vi "AWSEXE.vi"(8 "error in (no error)":errorcluster, 9 "New/Old(T)":bool, 10 "RX/RY":string, 11 "DUT":string) -> (0 "error in (out)":errorcluster, 2 "Result":string)   [LabVIEW 2024, in "AWSEXE.lvlib"]
doc: "This template is for the Queued Message Handler design pattern.\n\nThe Event Handling Loop generates messages based on user interface actions.\n\nThe Message Handling Loop processes messages generated by the Event Handling Loop, or by other messages. The messages are string values, so new messages can be added easily to the Message Cases case structure in the Message Handling Loop. Each message cluster can also provide an optional value for Message Data, which is a variant that can be converted to whatever message-specific data is required."
uses:
  AWSEXE.lvlib
  support/Neoway_ctrl.ctl
  controls/Neoway UI Data.ctl
  PrivateControls/FGV_Queue_Control.ctl
  <vilib>/Utility/error.llb/Error Cluster From Error Code.vi
  <vilib>/ErrorRing/Error Ring.xnode
  support/Message Queue/Neoway Message Queue.lvlib
  support/User Event - Stop/72-13360 User Event - Stop.lvlib
  Launcher/Launcher_DTU.lvlib
panel:
  in  "Neoway Flashing":T1
  in  "Config":string
  in  "Read_Res":bool
  in  "Read_Current":bool
  in  "Read_File":bool
  in  "Flash":bool
  out "queue name 2":string
  out "queue name":string
  out "Display <Replace Me>":string
  in  "Output":bool
  in  "Init_Neoway":bool
  in  "Exit":bool
  # "These controls have associated \"Value Changed\" events configured in the Event Structure on the diagram.\n\nReplace them (and reconfigure the Event Structure) with the controls you need for your application."
  # "This template is for the Queued Message Handler design pattern.\n\nSee the block diagram for more information on how to use this template."
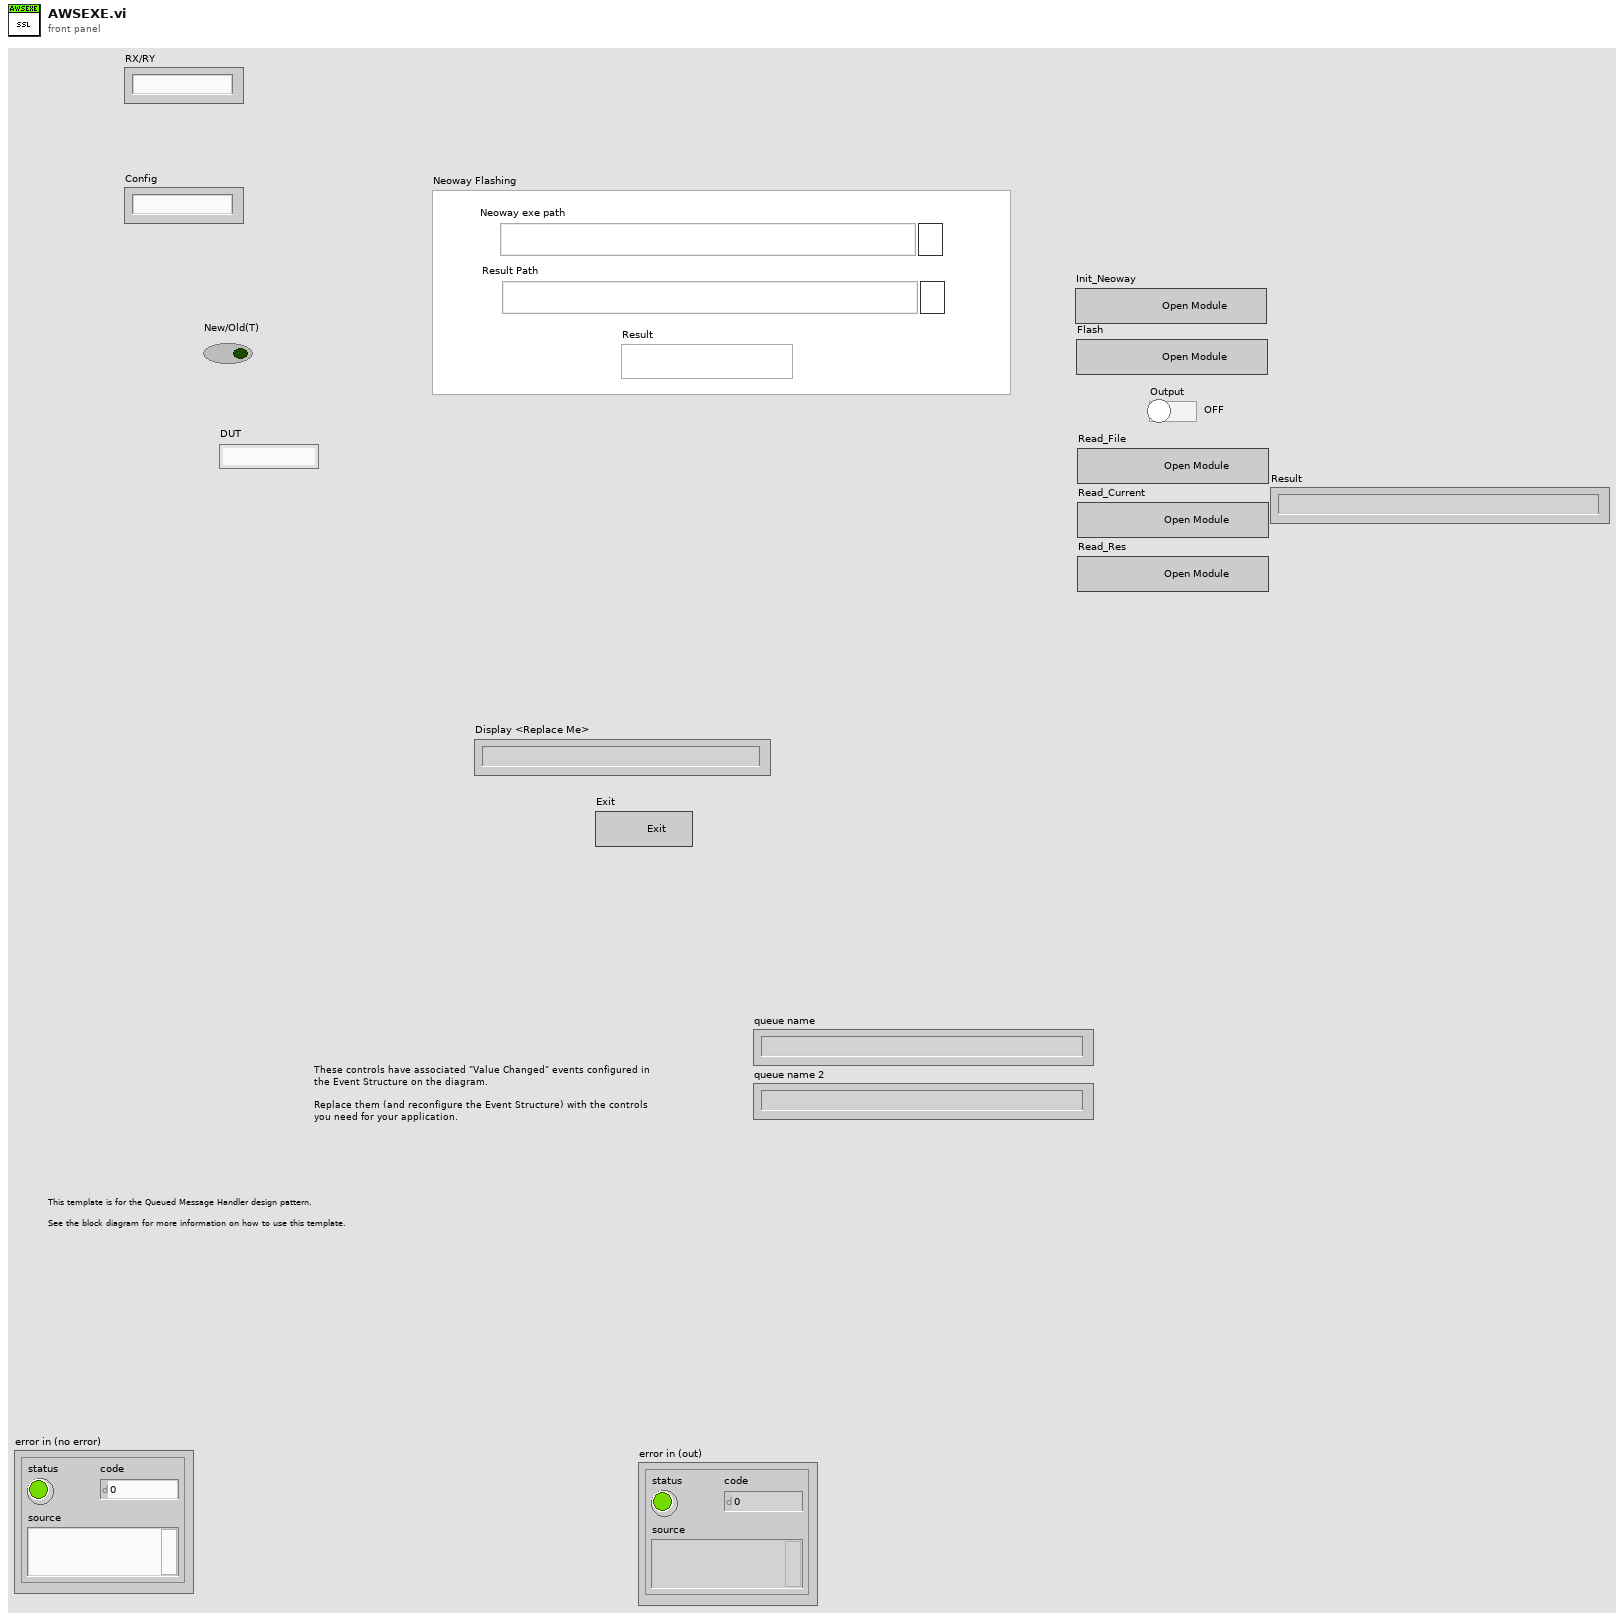
[diagram p1: front panel]
types:
  T1 = typedef "AWSEXE.lvlib/Neoway_ctrl.ctl" = cluster{"Neoway exe path":path, "Result Path":path, "Result":string}
  T2 = typedef "AWSEXE.lvlib/Neoway UI Data.ctl" = cluster{"DUT":string, "Neoway_Q":refnum<queue>, "notifier out":refnum<notifier>, "Config":string, "Neoway Flashing":T1, "Bat file path":path, "Exe path":string, "Flash path":string, "Result":string, "Timer":u32}
  T3 = typedef "AWSEXE.lvlib/FGV_Queue_Control.ctl" = enum16{"Release", "Get", "Set"}
  T4 = typedef "AWSEXE.lvlib/Neoway Message Queue.lvlib/All Message Queues.ctl" = cluster{"UI":refnum<queue>, "QSM":refnum<queue>}
  T5 = cluster{"Message":string, "Message Data":variant}
  T6 = enum16{"Read", "Write", "All_sections", "All_values", "Remove key&section"}
  T7 = enum16{"open", "replace", "create", "open or create", "replace or create", "replace or create with confirmation"}
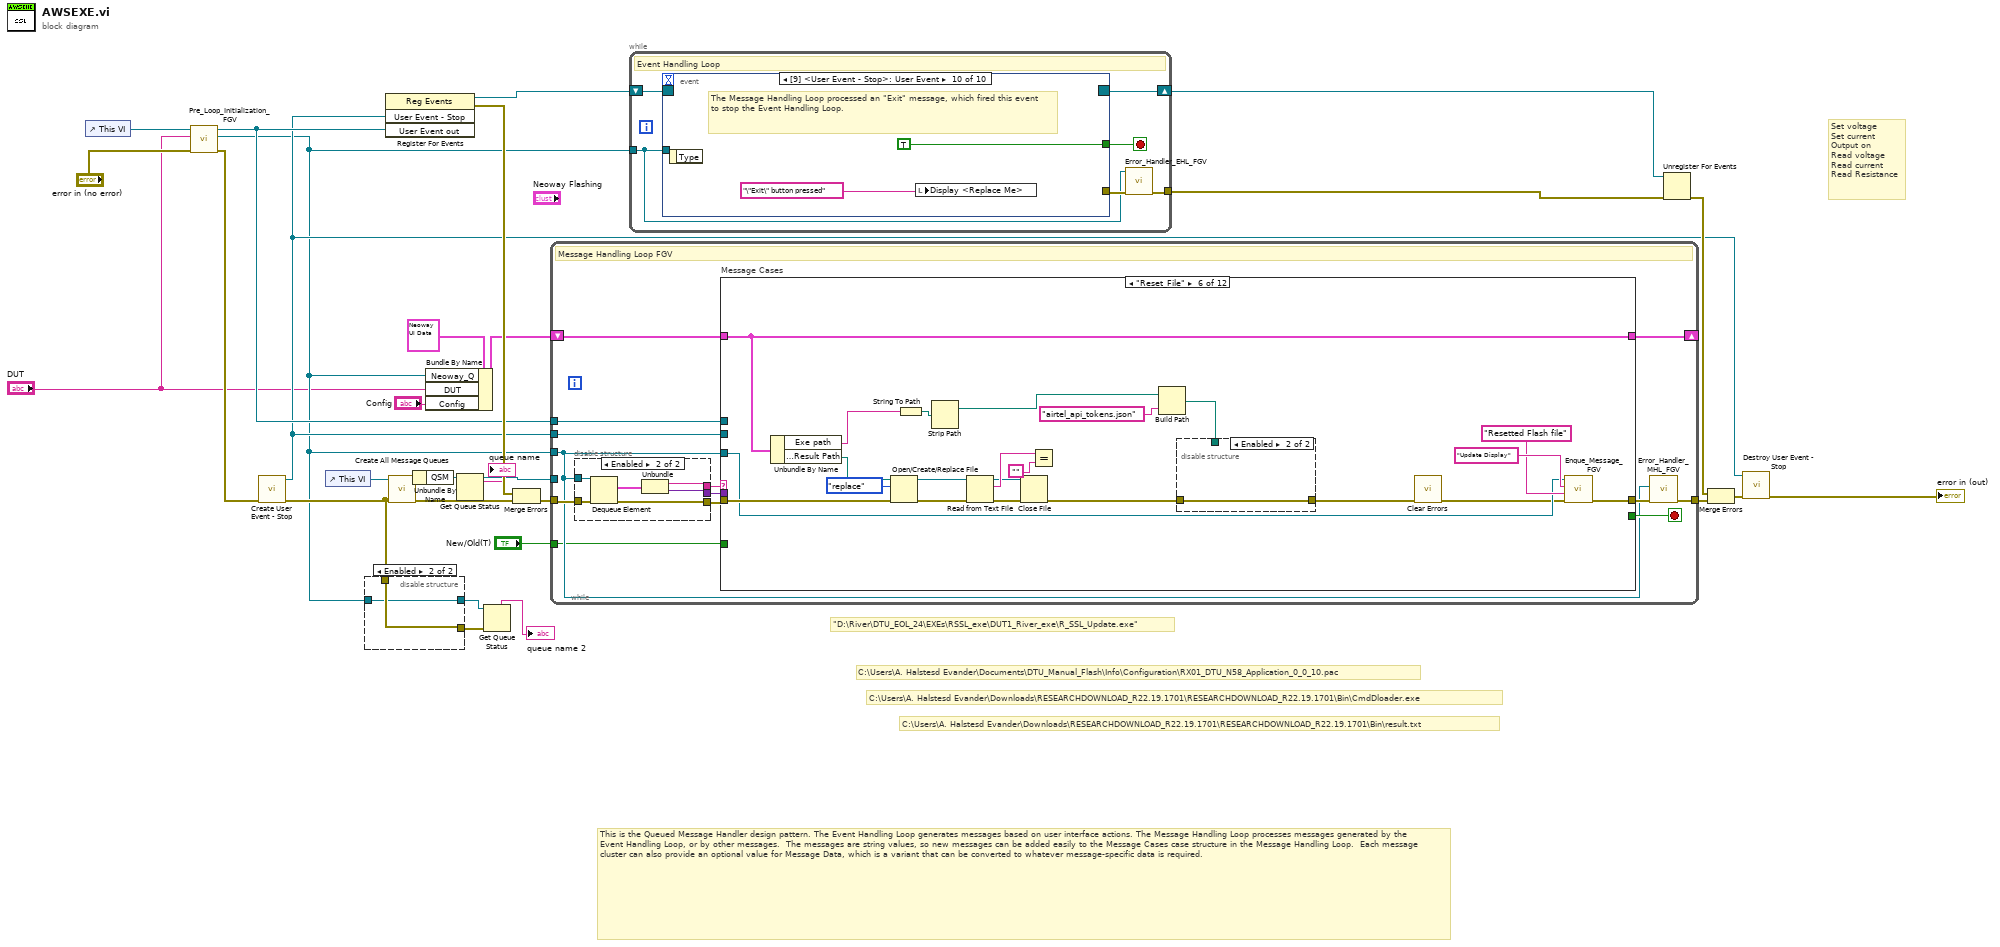
[diagram p0: block diagram]
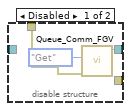
[diagram p2: hidden frame]
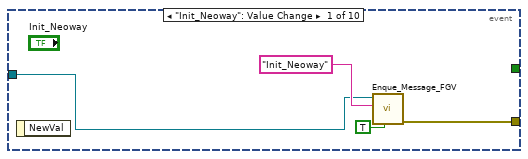
[diagram p3: hidden frame]
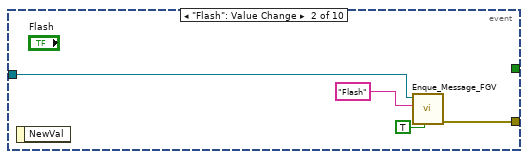
[diagram p4: hidden frame]
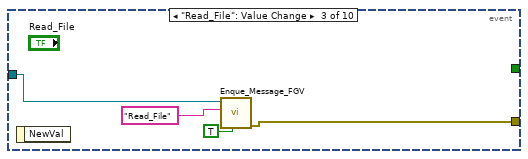
[diagram p5: hidden frame]
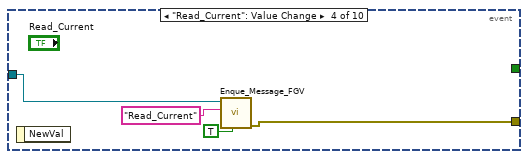
[diagram p6: hidden frame]
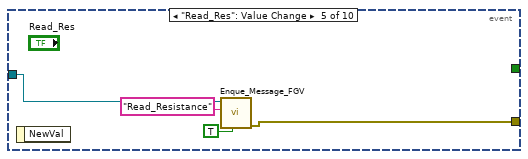
[diagram p7: hidden frame]
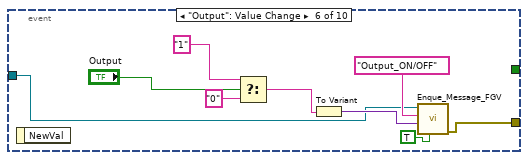
[diagram p8: hidden frame]
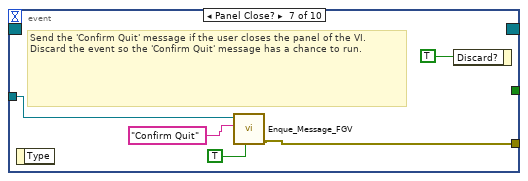
[diagram p9: hidden frame]
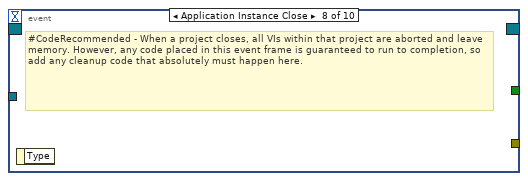
[diagram p10: hidden frame]
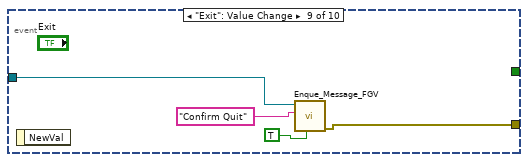
[diagram p11: hidden frame]
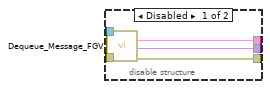
[diagram p12: hidden frame]
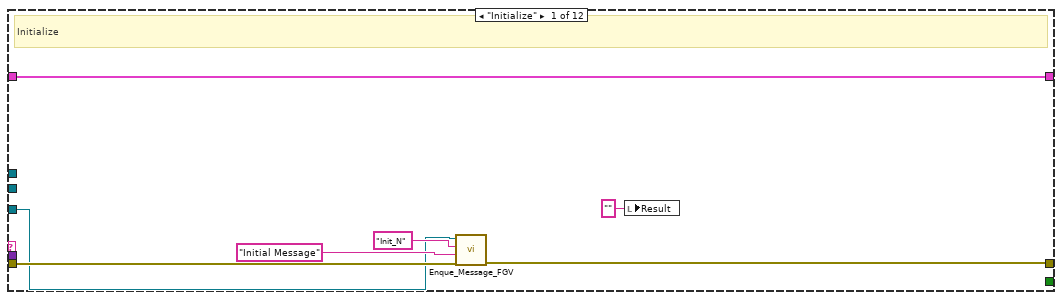
[diagram p13: hidden frame]
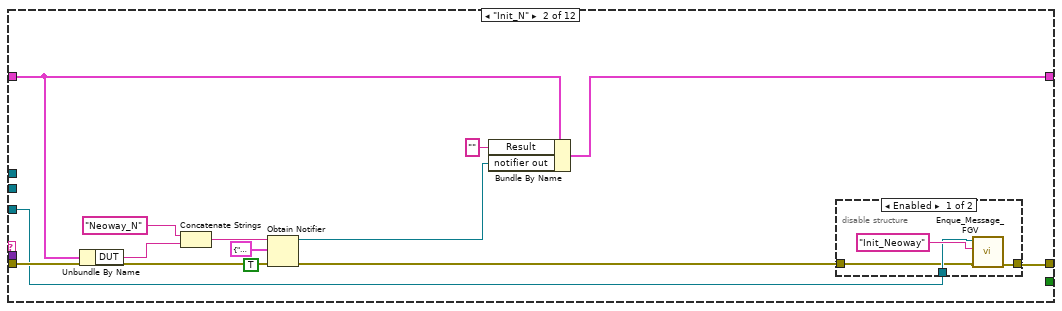
[diagram p14: hidden frame]
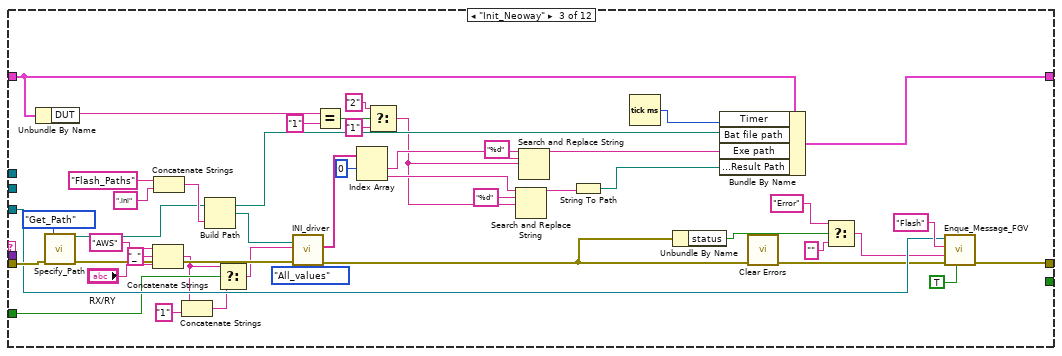
[diagram p16: hidden frame]
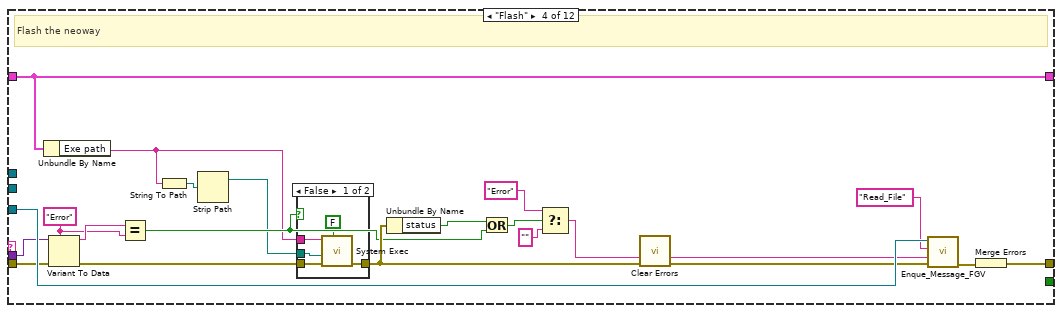
[diagram p17: hidden frame]
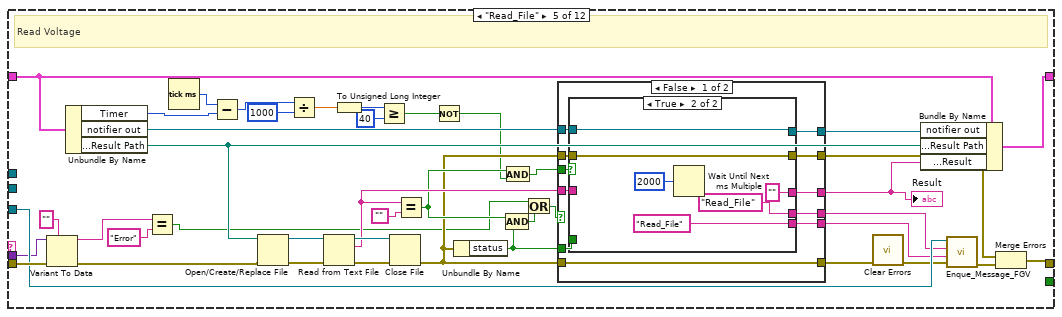
[diagram p19: hidden frame]
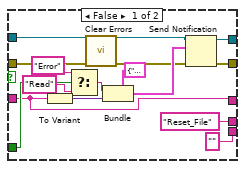
[diagram p20: hidden frame]
diagram:
  # "\"D:\\River\\DTU_EOL_24\\EXEs\\RSSL_exe\\DUT1_River_exe\\R_SSL_Update.exe\""
  # "C:\\Users\\A. Halstesd Evander\\Downloads\\RESEARCHDOWNLOAD_R22.19.1701\\RESEARCHDOWNLOAD_R22.19.1701\\Bin\\result.txt"
  # "C:\\Users\\A. Halstesd Evander\\Downloads\\RESEARCHDOWNLOAD_R22.19.1701\\RESEARCHDOWNLOAD_R22.19.1701\\Bin\\CmdDloader.exe"
  # "C:\\Users\\A. Halstesd Evander\\Documents\\DTU_Manual_Flash\\Info\\Configuration\\RX01_DTU_N58_Application_0_0_10.pac"
  # "Set voltage\nSet current\nOutput on\nRead voltage \nRead current\nRead Resistance"
  # "This is the Queued Message Handler design pattern. The Event Handling Loop generates messages based on user interface actions. The Message Handling Loop processes messages generated by the Event Handling Loop, or by other messages.  The messages are string values, so new messages can be added easily to the Message Cases case structure in the Message Handling Loop.  Each message cluster can also provide an optional value for Message Data, which is a variant that can be converted to whatever message-specific data is required."
  n1 = control-ref of="This VI"() -> (w18:refnum<vi>)
  n2 = call "Pre_Loop_Initialization_FGV.vi"("error in (no error)"="error in (no error)", "DUT"="DUT", "VI in"=w18) -> ("error out"=w16:errorcluster, "queue out"=w4:refnum<queue>, "User Event out"=w8:refnum<user-event>)  [unwired: 6 in]
  n3 = call "Create User Event - Stop.vi"("error in (no error)"=w16) -> ("error out"=w11:errorcluster, "User Event - Stop"=w7:refnum<user-event>)  [unwired: 9 in]
  n4 = control-ref of="This VI"() -> (w14:refnum<vi>)
  n5 = disable-structure shown="Enabled" {
    disable-tunnel: w11 -> [w33 w35]
    disable-tunnel: [w31 w34] -> w10
    disable-tunnel: [_ w35] -> w6
    disable-tunnel: w4 -> [_ w34]
    frame Disabled {
      n6 = call "Queue_Comm_FGV.vi"("error in (no error)"=w33, "Enum"=FGV_Queue_Control."Get") -> ("queue Out"=w31:refnum<queue>)  [unwired: 8 in, 1 out]
    }
    frame Enabled {
    }
  }
  n7 = register-events(w7, w8) -> (reference out=w21:refnum<event-registration>, error out=w19:errorcluster)  [unwired: 2 in]
  n8 = call "Create All Message Queues.vi"("error in (no error)"=w11, "This VI"=w14) -> ("error out"=w30:errorcluster, "Message Queues out"=w29:T4)  [unwired: 8 in]
  n9 = Unbundle By Name(w29) -> ("QSM"=w27:refnum<queue>)
  n10 = Bundle By Name(cluster=T2 {"DUT"="", "Neoway_Q"=refnum, "notifier out"=refnum, "Config"="", "Neoway Flashing"={"Neoway exe path"=path "", "Result Path"=path "", "Result"=""}, "Bat file path"=path "", "Exe path"="", "Flash path"="", "Result"="", "Timer"=0} ("Data Cluster"), "Neoway_Q"=w4, "DUT"="DUT", "Config"="Config") -> (w5:T2)
  n11 = Get Queue Status(queue=w27) -> (queue out=w13:refnum<queue>, queue name=→"queue name":string)  [unwired: 2 in, 6 out]
  n12 = Get Queue Status(queue=w10, error in (no error)=w6) -> (queue name=→"queue name 2":string)  [unwired: 1 in, 7 out]
  n13 = Merge Errors(w19, w30) -> (w20:errorcluster)
  n14 = while {
    tunnel: w13 -> [_]
    shift-right: [w47] -> _
    shift-left: w5 -> [w48]
    tunnel: w8 -> [w45]
    tunnel: w20 -> [w44]
    tunnel: [w39] -> w28
    tunnel: w7 -> [w38]
    tunnel: w4 -> [w37]
    tunnel: "New/Old(T)" -> [w36]
    stop <- w46 stop-if-true
    # "Message Handling Loop FGV"
    n15 = disable-structure shown="Enabled" {
      disable-tunnel: w44 -> [w52 w58]
      disable-tunnel: [w51 w56] -> w43
      disable-tunnel: [w50 w53] -> w42
      disable-tunnel: [w49 w54] -> w41
      disable-tunnel: w37 -> [_ w57]
      frame Disabled {
        n16 = call "Dequeue_Message_FGV.vi"("error in (no error)"=w52) -> ("error out"=w51:errorcluster, "Message Data"=w50:variant, "Message"=w49:string)  [unwired: 8 in]
      }
      frame Enabled {
        n17 = Dequeue Element(queue=w57, error in (no error)=w58) -> (element=w55:T5, error out=w56:errorcluster)  [unwired: 1 in, 2 out]
        n18 = Unbundle(w55) -> ("Message"=w54:string, "Message Data"=w53:variant)
      }
    }
    n19 = case "Message Cases" shown="\"Reset_File\"" w41 {
      selector: w41 -> [_ _ _ _ _ _ _ _ _ _ _ w320]
      tunnel: w43 -> [w61 w78 w128 w146 w197 w265 w280 w289 w298 w303 w311 _]
      tunnel: [w64 w67 w106 w149 w192 w252 w272 w287 w300 w301 w304 w321] -> w40
      tunnel: w48 -> [w65 w76 w114 w145 w195 w264 w281 w288 w295 w302 w306 w322]
      tunnel: [w65 w71 w119 w145 w194 w264 w281 w288 w295 w302 w306 w322] -> w47
      tunnel: [_ _ _ _ _ _ _ _ _ _ TRUE _] -> w46
      tunnel: w42 -> [_ _ _ w136 w191 _ w279 _ _ _ w313 _]
      tunnel: w45 -> [_ _ _ _ _ _ _ _ _ _ w314 _]
      tunnel: w38 -> [_ _ _ _ _ _ _ _ _ _ w309 _]
      tunnel: w37 -> [w60 w69 w105 w147 w193 w251 w271 w282 w293 _ w305 _]
      tunnel: w36 -> [_ _ w90 _ _ _ _ _ _ _ _ _]
      frame "Initialize" {
        # "Initialize"
        n20 = call "Enque_Message_FGV.vi"("error in (no error)"=w61, "Message Data"="Initial Message" ("Initial Message"), "Message"="Init_N", "queue in"=w60) -> ("error out"=w64:errorcluster)  [unwired: 7 in]
        n21 = local write "Result"("" ("Result")) -> ()
      }
      frame "Init_N" {
        n22 = Unbundle By Name(w76) -> ("DUT"=w75:string)
        n23 = Concatenate Strings("Neoway_N", w75) -> (w74:string)
        n24 = Obtain Notifier(name (unnamed)=w74, notification data type=T5 {"Message"="", "Message Data"=variant} ("notification"), create if not found? (T)=TRUE, error in (no error)=w78) -> (notifier out=w70:refnum<notifier>, error out=w68:errorcluster)  [unwired: 1 out]
        n25 = Bundle By Name(cluster=w76, "Result"="", "notifier out"=w70) -> (w71:T2)
        n26 = disable-structure shown="Enabled" {
          disable-tunnel: w69 -> [w81 _]
          disable-tunnel: w68 -> [w80 w83]
          disable-tunnel: [w79 w83] -> w67
          frame Enabled {
            n27 = call "Enque_Message_FGV.vi"("error in (no error)"=w80, "Message"="Init_Neoway", "queue in"=w81) -> ("error out"=w79:errorcluster)  [unwired: 8 in]
          }
          frame Disabled {
          }
        }
      }
      frame "Init_Neoway" {
        n28 = Unbundle By Name(w114) -> ("DUT"=w85:string)
        n29 = call "Specify_Path.vi"("Path_Enum"=enum16{"Find_Path", "Get_Path"}."Get_Path", "error in (no error)"=w128) -> ("Configurations"=w117:path, "error out"=w123:errorcluster)  [unwired: 6 in, 6 out]
        n30 = Concatenate Strings("AWS" ("Section"), "_" ("string"), "RX/RY") -> (w88:string)
        n31 = Concatenate Strings("Flash_Paths" ("string"), ".ini" ("string")) -> (w125:string)
        n32 = Concatenate Strings(w88, "1" ("string")) -> (w89:string)
        n33 = Build Path(base path=w117, name or relative path=w125) -> (appended path=w124:path)
        n34 = Select(t=w88, s=w90, f=w89) -> (s? t:f=w86:string)
        n35 = call "INI_driver.vi"("Enum"=T6."All_values", "instrument file path"=w124, "error in (no error)"=w123, "Section"=w86) -> ("error out"=w101:errorcluster, "Values out"=w121:string[])  [unwired: 4 in, 2 out]
        n36 = Equal?(x=w85, y="1") -> (x = y?=w96:bool)
        n37 = Index Array(array=w121, index #1=0 ("index")) -> (element #1=w116:string, element #2=w111:string)  [unwired: 1 in]
        n38 = Select(t="2" ("y"), s=w96, f="1") -> (s? t:f=w84:string)
        n39 = Search and Replace String(input string=w111, search string="%d", replace string=w84) -> (result string=w110:string)  [unwired: 5 in, 3 out]
        n40 = Search and Replace String(input string=w116, search string="%d", replace string=w84) -> (result string=w113:string)  [unwired: 5 in, 3 out]
        n41 = String To Path(string=w110) -> (path=w109:path)
        n42 = Tick Count (ms)() -> (millisecond timer value=w98:u32)
        n43 = Unbundle By Name(w101) -> ("status"=w103:bool)
        n44 = Bundle By Name(cluster=w114, "Timer"=w98, "Bat file path"=w117, "Exe path"=w113, "Neoway Flashing.Result Path"=w109) -> (w119:T2)
        n45 = call <vilib>:"Clear Errors.vi"("error in (no error)"=w101) -> ("error out"=w99:errorcluster)  [unwired: 5 in, 1 out]
        n46 = Select(t="Error" ("\"Do Something\" button pressed"), s=w103, f="" ("\"Do Something\" button pressed")) -> (s? t:f=w100:string)
        n47 = call "Enque_Message_FGV.vi"("Priority"=TRUE ("Priority Message? (F)"), "error in (no error)"=w99, "Message Data"=w100, "Message"="Flash", "queue in"=w105) -> ("error out"=w106:errorcluster)  [unwired: 6 in]
      }
      frame "Flash" {
        w133 = "Error" ("Message")
        # "Flash the neoway"
        n48 = Unbundle By Name(w145) -> ("Exe path"=w131:string)
        n49 = Variant To Data(error in=w146, type=w133, Variant=w136) -> (data=w134:string, error out=w137:errorcluster)
        n50 = Equal?(x=w134, y=w133) -> (x = y?=w132:bool)
        n51 = String To Path(string=w131) -> (path=w130:path)
        n52 = Strip Path(path=w130) -> (stripped path=w129:path)  [unwired: 1 out]
        n53 = case shown="False" w132 {
          tunnel: w131 -> [w154 _]
          tunnel: [w153 w155] -> w144
          tunnel: w137 -> [w152 w155]
          tunnel: w129 -> [w150 _]
          frame False {
            n54 = call <vilib>:"System Exec.vi"("wait until completion? (T)"=FALSE, "error in (no error)"=w152, "working directory"=w150, "command line"=w154) -> ("error out"=w153:errorcluster)  [unwired: 4 in, 3 out]
          }
          frame True {
          }
        }
        n55 = Unbundle By Name(w144) -> ("status"=w141:bool)
        n56 = Or(x=w141, y=w132) -> (x .or. y?=w135:bool)
        n57 = Select(t="Error" ("\"Do Something\" button pressed"), s=w135, f="" ("\"Do Something\" button pressed")) -> (s? t:f=w139:string)
        n58 = call <vilib>:"Clear Errors.vi"("error in (no error)"=w144) -> ("error out"=w138:errorcluster)  [unwired: 5 in, 1 out]
        n59 = call "Enque_Message_FGV.vi"("error in (no error)"=w138, "Message Data"=w139, "Message"="Read_File", "queue in"=w147) -> ("error out"=w148:errorcluster)  [unwired: 7 in]
        n60 = Merge Errors(w148) -> (w149:errorcluster)
      }
      frame "Read_File" {
        # "Read Voltage"
        n61 = Variant To Data(error in=w197, type="", Variant=w191) -> (data=w188:string, error out=w187:errorcluster)
        n62 = Unbundle By Name(w195) -> ("Timer"=w165:u32, "notifier out"=w178:refnum<notifier>, "Neoway Flashing.Result Path"=w181:path)
        n63 = Equal?(x=w188, y="Error" ("\"Do Something\" button pressed")) -> (x = y?=w169:bool)
        n64 = Tick Count (ms)() -> (millisecond timer value=w166:u32)
        n65 = Subtract(x=w166, y=w165) -> (x-y=w164:u32)
        n66 = Open/Create/Replace File(file path (use dialog)=w181, error in=w187) -> (refnum out=w184:refnum<file>, error out=w186:errorcluster)  [unwired: 4 in, 1 out]
        n67 = Divide(x=w164, y=u32 1000) -> (x/y=w162:dbl)
        n68 = Read from Text File(file (use dialog)=w184, error in=w186) -> (refnum out=w182:refnum<file>, text=w176:string, error out=w185:errorcluster)  [unwired: 2 in, 1 out]
        n69 = To Unsigned Long Integer(number=w162) -> (unsigned 32bit integer=w161:u32)
        n70 = Greater Or Equal?(x=w161, y=u32 40) -> (x >= y?=w158:bool)
        n71 = Close File(refnum=w182, error in=w185) -> (error out=w171:errorcluster)  [unwired: 1 out]
        n72 = Equal?(x=w176, y="") -> (x = y?=w174:bool)
        n73 = Not(x=w158) -> (.not. x?=w156:bool)
        n74 = Unbundle By Name(w171) -> ("status"=w175:bool)
        n75 = And(x=w174, y=w156) -> (x .and. y?=w159:bool)
        n76 = Compound Arithmetic op=AND(w174, w175) -> (w168:bool)
        n77 = Or(x=w169, y=w168) -> (x .or. y?=w167:bool)
        n78 = case shown="False" w167 {
          tunnel: w171 -> [w208 w235]
          tunnel: [w207 w236] -> w179
          tunnel: w178 -> [w206 w238]
          tunnel: [w205 w237] -> w177
          tunnel: w176 -> [w204 _]
          tunnel: w175 -> [w203 _]
          tunnel: w159 -> [w202 _]
          tunnel: [w201 "Reset_File" ("Message")] -> w173
          tunnel: [w200 "" ("\"Do Something\" button pressed")] -> w172
          tunnel: w171 -> [w199 w243]
          tunnel: [w199 w243] -> w170
          tunnel: [w198 ""] -> w157
          frame False {
            n79 = case shown="True" w202 {
              tunnel: w208 -> [w217 w225]
              tunnel: [w215 w225] -> w207
              tunnel: w206 -> [w214 w229]
              tunnel: [w213 w229] -> w205
              tunnel: w204 -> [w209 _]
              tunnel: w203 -> [w212 _]
              tunnel: ["Reset_File" ("Message") "Read_File" ("Message")] -> w201
              tunnel: ["" ("\"Do Something\" button pressed") "Read_File" ("\"Do Something\" button pressed")] -> w200
              tunnel: [w209 ""] -> w198
              frame False {
                n80 = To Variant(anything=w209) -> (Variant=w222:variant)
                n81 = Select(t="Error" ("f"), s=w212, f="Read" ("Message")) -> (s? t:f=w223:string)
                n82 = call <vilib>:"Clear Errors.vi"("error in (no error)"=w217) -> ("error out"=w216:errorcluster)  [unwired: 5 in, 1 out]
                n83 = Bundle(cluster=T5 {"Message"="", "Message Data"=variant} ("notification"), "Message"=w223, "Message Data"=w222) -> (w221:T5)
                n84 = Send Notification(notification=w221, notifier=w214, error in (no error)=w216) -> (notifier out=w213:refnum<notifier>, error out=w215:errorcluster)
              }
              frame True {
                n85 = Wait Until Next ms Multiple(millisecond multiple=u32 2000) -> ()  [unwired: 1 out]
              }
            }
          }
          frame True {
            n86 = To Variant(anything=errorcluster {"status"=TRUE, "code"=0, "source"="Error at N58 Flashing"} ("error constant")) -> (Variant=w242:variant)
            n87 = call <vilib>:"Clear Errors.vi"("error in (no error)"=w235) -> ("error out"=w239:errorcluster)  [unwired: 5 in, 1 out]
            n88 = Bundle(cluster=T5 {"Message"="", "Message Data"=variant} ("notification"), "Message"="Error" ("f"), "Message Data"=w242) -> (w241:T5)
            n89 = Send Notification(notification=w241, notifier=w238, error in (no error)=w239) -> (notifier out=w237:refnum<notifier>, error out=w236:errorcluster)
          }
        }
        "Result" <- w157
        n90 = call <vilib>:"Clear Errors.vi"("error in (no error)"=w170) -> ("error out"=w180:errorcluster)  [unwired: 5 in, 1 out]
        n91 = Bundle By Name(cluster=w195, "notifier out"=w177, "Neoway Flashing.Result Path"=w181, "Neoway Flashing.Result"=w157) -> (w194:T2)
        n92 = call "Enque_Message_FGV.vi"("error in (no error)"=w180, "Message Data"=w172, "Message"=w173, "queue in"=w193) -> ("error out"=w196:errorcluster)  [unwired: 7 in]
        n93 = Merge Errors(w179, w196) -> (w192:errorcluster)
      }
      frame "Reset_File" {
        n94 = Unbundle By Name(w264) -> ("Exe path"=w249:string, "Neoway Flashing.Result Path"=w262:path)
        n95 = Open/Create/Replace File(file path (use dialog)=w262, error in=w265, operation (0:open)=T7."replace") -> (refnum out=w259:refnum<file>, error out=w263:errorcluster)  [unwired: 3 in, 1 out]
        n96 = String To Path(string=w249) -> (path=w250:path)
        n97 = Strip Path(path=w250) -> (stripped path=w247:path)  [unwired: 1 out]
        n98 = Read from Text File(file (use dialog)=w259, error in=w263) -> (refnum out=w256:refnum<file>, text=w257:string, error out=w260:errorcluster)  [unwired: 2 in, 1 out]
        n99 = Close File(refnum=w256, error in=w260) -> (error out=w253:errorcluster)  [unwired: 1 out]
        n100 = Equal?(x=w257, y="") -> ()  [unwired: 1 out]
        n101 = Build Path(base path=w247, name or relative path="airtel_api_tokens.json") -> (appended path=w245:path)
        n102 = disable-structure shown="Enabled" {
          disable-tunnel: w253 -> [w269 w270]
          disable-tunnel: [w268 w270] -> w246
          disable-tunnel: w245 -> [w267 _]
          frame Disabled {
            n103 = Delete(path (use dialog)=w267, confirm (F)=FALSE, error in=w269) -> (error out=w268:errorcluster)  [unwired: 2 in, 2 out]
          }
          frame Enabled {
          }
        }
        n104 = call <vilib>:"Clear Errors.vi"("error in (no error)"=w246) -> ("error out"=w244:errorcluster)  [unwired: 5 in, 1 out]
        n105 = call "Enque_Message_FGV.vi"("error in (no error)"=w244, "Message Data"="Resetted Flash file" ("\"Do Something\" button pressed"), "Message"="Update Display", "queue in"=w251) -> ("error out"=w252:errorcluster)  [unwired: 7 in]
      }
      frame "Update Display" {
        # "#CodeRecommended - If you wish to decouple the Message Handling Loop from your user interface, consider creating User Events (like the \"Stop\" event in this VI) to message the Event Handling Loop whenever the user interface needs updating."
        # "Update Display - Convert the message data to a string to display in the Data Display indicator."
        n106 = Variant To Data(error in=w280, type="", Variant=w279) -> (data=→"Display <Replace Me>":string, error out=w277:errorcluster)
        n107 = call <vilib>:"Clear Errors.vi"("error in (no error)"=w277) -> ("error out"=w275:errorcluster)  [unwired: 5 in, 1 out]
        n108 = Merge Errors(w275) -> (w273:errorcluster)
        n109 = call "Enque_Message_FGV.vi"("error in (no error)"=w273, "Message"="Confirm Quit", "queue in"=w271) -> ("error out"=w272:errorcluster)  [unwired: 8 in]
      }
      frame "Error" {
        # "Error - Display an error dialog. This message is sent by the \"Error Handler\" VIs at the end of other loops in this application."
        n110 = call <vilib>:"Clear Errors.vi"("error in (no error)"=w289) -> ("error out"=w284:errorcluster)  [unwired: 5 in, 1 out]
        n111 = call "Enque_Message_FGV.vi"("Priority"=TRUE ("Priority Message? (F)"), "error in (no error)"=w284, "Message"="Confirm Quit", "queue in"=w282) -> ("error out"=w283:errorcluster)  [unwired: 7 in]
        n112 = Merge Errors(w283) -> (w287:errorcluster)
      }
      frame "Confirm Quit" {
        # "Confirm Quit - Message that can confirm whether or not the user wants to exit the application."
        n113 = Unbundle By Name(w295) -> ("notifier out"=w291:refnum<notifier>)
        n114 = Release Notifier(notifier=w291, force destroy? (F)=TRUE, error in (no error)=w298) -> (error out=w292:errorcluster)  [unwired: 2 out]
        n115 = call <vilib>:"Clear Errors.vi"("error in (no error)"=w292) -> ("error out"=w294:errorcluster)  [unwired: 5 in, 1 out]
        n116 = call "Enque_Message_FGV.vi"("Priority"=TRUE ("Priority Message? (F)"), "error in (no error)"=w294, "Message"="Exit", "queue in"=w293) -> ("error out"=w299:errorcluster)  [unwired: 7 in]
        n117 = Merge Errors(w299) -> (w300:errorcluster)
      }
      frame "---Copy This Frame---" {
        # "Duplicate this frame when creating new messages.  Change this comment in the duplicated frame to describe this message."
        n118 = Merge Errors(w303) -> (w301:errorcluster)
      }
      frame "Exit" {
        # "Stop the VI"
        # "Release the message queue reference"
        # "Exit - Exit the application."
        n119 = disable-structure shown="Enabled" {
          disable-tunnel: w313 -> [w317 _]
          frame Disabled {
            n120 = Variant To Data(type=errorcluster {"status"=FALSE, "code"=0, "source"=""} ("error constant"), Variant=w317) -> (data=w318:errorcluster)  [unwired: 1 in, 1 out]
            n121 = call <vilib>:"Simple Error Handler.vi"("error in (no error)"=w318) -> ()  [unwired: 4 in, 5 out]
          }
          frame Enabled {
          }
        }
        n122 = call "Queue_Comm_FGV.vi"("error in (no error)"=w311, "Enum"=FGV_Queue_Control."Release", "queue in"=w305) -> ("error Out"=w310:errorcluster)  [unwired: 7 in, 1 out]
        n123 = call "Fire User Event - Stop.vi"("User Event - Stop"=w309) -> ("error out"=w307:errorcluster)  [unwired: 10 in]
        n124 = call "Fire User Event - Stop.vi"("User Event - Stop"=w314) -> ("error out"=w308:errorcluster)  [unwired: 10 in]
        n125 = Merge Errors(w308, w307, w310) -> (w315:errorcluster)
        n126 = call <vilib>:"Clear Errors.vi"("error in (no error)"=w315) -> ("error out"=w304:errorcluster)  [unwired: 5 in, 1 out]
      }
      frame Default {
        # "'Default' case only runs if there is a message that isn't defined in any of the other cases.  Output a programming error."
        n127 = xnode "Error Ring"("parameter 0"=w320) -> ("error out"=w321:errorcluster)
      }
    }
    n128 = call "Error_Handler_MHL_FGV.vi"("error in (no error)"=w40, "queue in"=w37) -> ("error Out"=w39:errorcluster)  [unwired: 9 in]
  }
  n129 = while {
    shift-right: [w334] -> w24
    shift-left: w21 -> [w335]
    tunnel: [w331] -> w22
    tunnel: w4 -> [w330]
    stop <- w333 stop-if-true
    # "Event Handling Loop"
    n130 = event shown="[9] <User Event - Stop>: User Event" {
      selector: w335 -> [_ _ _ _ _ _ _ _ _ _]
      dyn-events: [_ _ _ _ _ _ _ _ _ _] -> w334
      timeout: _ -> [_ _ _ _ _ _ _ _ _ _]
      tunnel: [_ _ _ _ _ _ _ _ _ TRUE ("Discard?")] -> w333
      tunnel: [w338 w342 w346 w350 w354 w362 w368 _ w373 _] -> w332
      tunnel: w330 -> [w336 w340 w344 w348 w352 w356 w365 _ w370 _]
      event "Init_Neoway": Value Change {
        n131 = event-data() -> ()  [unwired: 1 in, 1 out]
        n132 = call "Enque_Message_FGV.vi"("Priority"=TRUE ("Priority Message? (F)"), "Message"="Init_Neoway", "queue in"=w336) -> ("error out"=w338:errorcluster)  [unwired: 8 in]
      }
      event "Flash": Value Change {
        n133 = event-data() -> ()  [unwired: 1 in, 1 out]
        n134 = call "Enque_Message_FGV.vi"("Priority"=TRUE ("Priority Message? (F)"), "Message"="Flash", "queue in"=w340) -> ("error out"=w342:errorcluster)  [unwired: 8 in]
      }
      event "Read_File": Value Change {
        n135 = event-data() -> ()  [unwired: 1 in, 1 out]
        n136 = call "Enque_Message_FGV.vi"("Priority"=TRUE ("Priority Message? (F)"), "Message"="Read_File", "queue in"=w344) -> ("error out"=w346:errorcluster)  [unwired: 8 in]
      }
      event "Read_Current": Value Change {
        n137 = event-data() -> ()  [unwired: 1 in, 1 out]
        n138 = call "Enque_Message_FGV.vi"("Priority"=TRUE ("Priority Message? (F)"), "Message"="Read_Current", "queue in"=w348) -> ("error out"=w350:errorcluster)  [unwired: 8 in]
      }
      event "Read_Res": Value Change {
        n139 = event-data() -> ()  [unwired: 1 in, 1 out]
        n140 = call "Enque_Message_FGV.vi"("Priority"=TRUE ("Priority Message? (F)"), "Message"="Read_Resistance", "queue in"=w352) -> ("error out"=w354:errorcluster)  [unwired: 8 in]
      }
      event "Output": Value Change {
        n141 = event-data() -> ()  [unwired: 1 in, 1 out]
        n142 = Select(t="1", s="Output", f="0") -> (s? t:f=w358:string)
        n143 = To Variant(anything=w358) -> (Variant=w357:variant)
        n144 = call "Enque_Message_FGV.vi"("Priority"=TRUE ("Priority Message? (F)"), "Message Data"=w357, "Message"="Output_ON/OFF", "queue in"=w356) -> ("error out"=w362:errorcluster)  [unwired: 7 in]
      }
      event Panel Close? {
        # "Send the 'Confirm Quit' message if the user closes the panel of the VI. Discard the event so the 'Confirm Quit' message has a chance to run."
        n145 = event-data() -> ()  [unwired: 1 in, 1 out]
        n146 = call "Enque_Message_FGV.vi"("Priority"=TRUE ("Priority Message? (F)"), "Message"="Confirm Quit", "queue in"=w365) -> ("error out"=w368:errorcluster)  [unwired: 8 in]
        n147 = event-data("Discard?"=TRUE) -> ()  [unwired: 1 in, 1 out]
      }
      event Application Instance Close {
        # "#CodeRecommended - When a project closes, all VIs within that project are aborted and leave memory. However, any code placed in this event frame is guaranteed to run to completion, so add any cleanup code that absolutely must happen here."
        n148 = event-data() -> ()  [unwired: 1 in, 1 out]
      }
      event "Exit": Value Change {
        n149 = event-data() -> ()  [unwired: 1 in, 1 out]
        n150 = call "Enque_Message_FGV.vi"("Priority"=TRUE ("Priority Message? (F)"), "Message"="Confirm Quit", "queue in"=w370) -> ("error out"=w373:errorcluster)  [unwired: 8 in]
      }
      event User Event {
        # "The Message Handling Loop processed an \"Exit\" message, which fired this event to stop the Event Handling Loop."
        n151 = event-data() -> ()  [unwired: 1 in, 1 out]
        n152 = local write "Display <Replace Me>"("\"Exit\" button pressed" ("VI Stopped")) -> ()
      }
    }
    n153 = call "Error_Handler_EHL_FGV.vi"("error in (no error)"=w332, "queue in"=w330) -> ("error Out"=w331:errorcluster)  [unwired: 9 in]
  }
  n154 = Unregister For Events(event registration refnum=w24, error in=w22) -> (error out=w25:errorcluster)
  n155 = Merge Errors(w25, w28) -> (w26:errorcluster)
  n156 = call "Destroy User Event - Stop.vi"("error in (no error)"=w26, "User Event - Stop"=w7) -> ("error out"=→"error in (out)":errorcluster)  [unwired: 9 in]
